vi "Required Buffer Size (Transfer).vi"(8 "error in (no error)":errorcluster, 11 "Transfer Configuration in":T1 {"channels"."dst buffer offset" format="%d bytes"; "channels"."src buffer offset" format="%d bytes"}) -> (0 "error out":errorcluster, 2 "required buffer size":u64 format="%d bytes", 3 "Transfer Configuration out":T1 {"channels"."dst buffer offset" format="%d bytes"; "channels"."src buffer offset" format="%d bytes"})   [LabVIEW 2017, in "DSF Core.lvlib"]
uses:
  DSF Core.lvlib
  Controls/DSF Engine Transfer Configuration.ctl
  Controls/DSF Byte Order.ctl
  Controls/DSF Engine Channel Configuration.ctl
  Controls/DSF Data Type.ctl
  Controls/DSF Settings Info.ctl
  Shared/VIs/Sizeof.vi
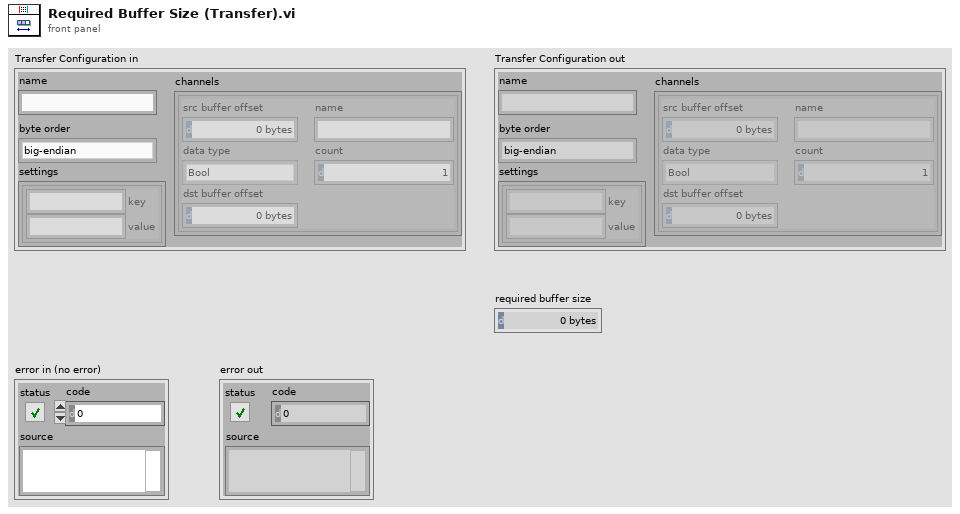
[diagram p1: front panel]
types:
  T1 = typedef "DSF Core.lvlib/DSF Engine Transfer Configuration.ctl" = cluster{"name":string, "byte order":T2, "channels":T3[], "settings":T5}
  T2 = typedef "DSF Core.lvlib/DSF Byte Order.ctl" = enum8{"big-endian", "little-endian"}
  T3 = typedef "DSF Core.lvlib/DSF Engine Channel Configuration.ctl" = cluster{"src buffer offset":u64, "name":string, "data type":T4, "count":u64, "dst buffer offset":u64}
  T4 = typedef "DSF Core.lvlib/DSF Data Type.ctl" = enum8{"Bool", "SGL", "DBL", "I8", "I16", "I32", "I64", "U8", "U16", "U32", "U64"}
  T5 = typedef "DSF Core.lvlib/DSF Settings Info.ctl" = cluster{"key":string, "value":string}[]
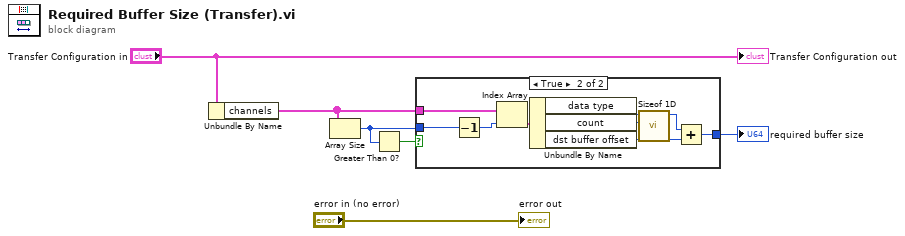
[diagram p0: block diagram]
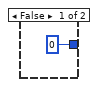
[diagram p2: hidden frame]
diagram:
  n1 = Unbundle By Name("Transfer Configuration in") -> ("channels"=w3:T3[])
  n2 = Array Size(array=w3) -> (size(s)=w6:i32)
  n3 = Greater Than 0?(x=w6) -> (x > 0?=w5:bool)
  n4 = case shown="True" w5 {
    tunnel: w6 -> [_ w16]
    tunnel: w3 -> [_ w15]
    tunnel: [u64 0 w8] -> w4
    frame False {
    }
    frame True {
      n5 = Decrement(x=w16) -> (x-1=w14:i32)
      n6 = Index Array(array=w15, index=w14) -> (element=w13:T3)
      n7 = Unbundle By Name(w13) -> ("data type"=w12:T4, "count"=w11:u64, "dst buffer offset"=w10:u64)
      n8 = call "Sizeof 1D.vi"("count"=w11, "data type"=w12) -> ("size in bytes"=w9:u64)  [unwired: 9 in]
      n9 = Add(x=w9, y=w10) -> (x+y=w8:u64)
    }
  }
  "required buffer size" <- w4
  "Transfer Configuration out" <- "Transfer Configuration in"
  "error out" <- "error in (no error)"
